vi "Send Create Room Service Request.vi"(7 "Message Priority (Normal)":T1=enum."Normal", 8 "error in (no error)":errorcluster, 9 "Room Service":refnum<class "Room Service Base.lvclass">, 10 "Rooms No":string, 11 "Message Enqueuer":refnum<class "Message Enqueuer.lvclass">) -> (0 "error out":errorcluster, 3 "Message Enqueuer out":refnum<class "Message Enqueuer.lvclass">)   [LabVIEW 2023, in "Incoming Hotel Management Tool Model Interface.lvlib" / "Create Room Service Request Msg.lvclass"]
doc: "This VI sends the message to an actor."
uses:
  Create Room Service Request Msg.lvclass
  Create Room Service Request Msg.lvclass/Create Room Service Request Msg.ctl
  <vilib>/ActorFramework/Message Enqueuer/Message Enqueuer.lvclass
  C:/Program Files/National Instruments/LabVIEW 2023/vi.lib/ActorFramework/Message/Message.lvclass
  C:/Users/bhaghyaraj/Trainings/NI Actor Framework/SDLC/Interfaces/Incoming Hotel Management Tool Model Interface Messages/Create Room Service Request Msg/Create Room Service Request Msg.lvclass
  <vilib>/ActorFramework/Message Enqueuer/Message Priority.ctl
  Room Service Types/Room Service Base/Room Service Base.lvclass
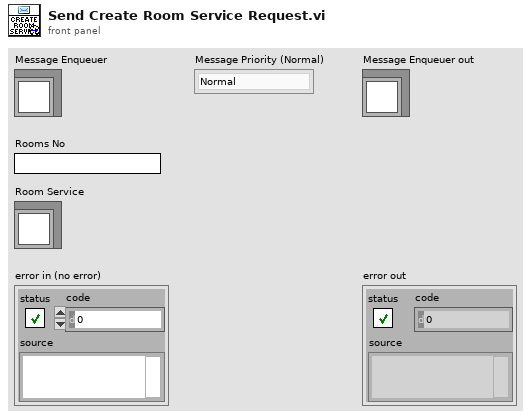
[diagram p1: front panel]
types:
  T1 = typedef "Actor Framework.lvlib/Message Enqueuer.lvclass/Message Priority.ctl" = enum16{"Low", "Normal", "High"}
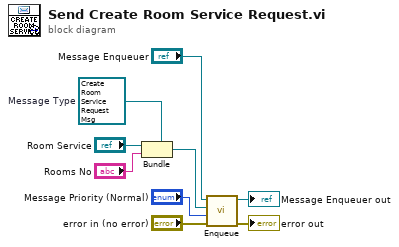
[diagram p0: block diagram]
diagram:
  w6 = refnum<class "Create Room Service Request Msg.lvclass"> refnum  # Message Type
  n1 = Bundle(cluster=w6, "Room Service", "Rooms No") -> (w5:refnum<class "Create Room Service Request Msg.lvclass">)
  n2 = call <vilib>:"Enqueue.vi"("error in (no error)"="error in (no error)", "Message Priority (Normal)"="Message Priority (Normal)", "Message"=w5, "Message Enqueuer in"="Message Enqueuer") -> ("error out"=→"error out":errorcluster, "Message Enqueuer out"=→"Message Enqueuer out":refnum<class "Message Enqueuer.lvclass">)  [unwired: 6 in]
